vi "Connect.vi"(8 "error in (no error)":errorcluster, 10 "Session - Pipeline":path=path "Z:/users/Manolis/Labview/Scanner/sessions.dsn", 11 "Database in":refnum<class "Database.lvclass">) -> (0 "error out":errorcluster, 3 "Database out":refnum<class "Database.lvclass">)   [LabVIEW 2014, in "Database.lvclass"]
uses:
  Database.lvclass
  Database.lvclass/Database.ctl
  <vilib>/addons/database/Connection.llb/DB Tools Open Connec (Path).vi
  <vilib>/addons/database/NI_Database_API.lvlib
panel:
  in  "Session - Commons":path=path "Z:/users/Manolis/Labview/Scanner/sessions.dsn"
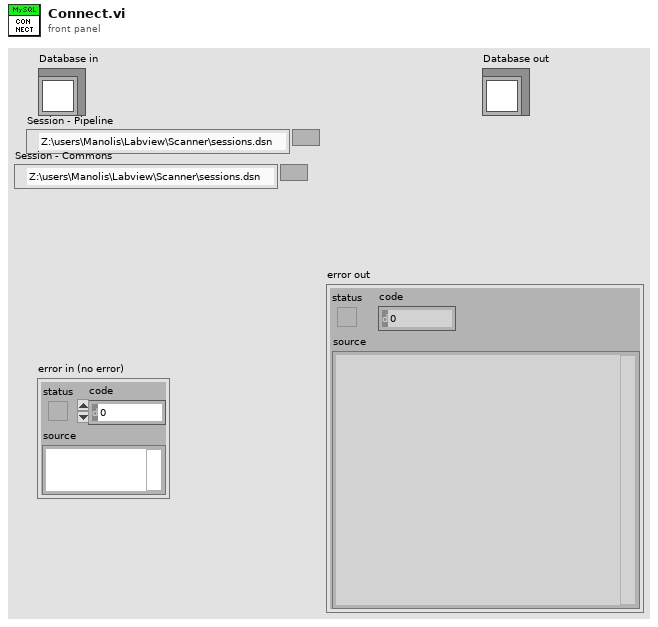
[diagram p1: front panel]
types:
  T1 = typedef "NI_Database_API.lvlib/Conn ObjectReference.ctl" = refnum<k1>
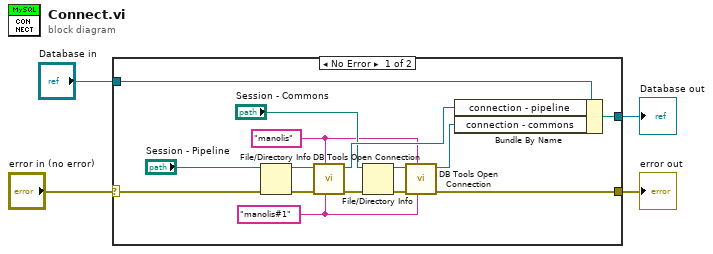
[diagram p0: block diagram]
diagram:
  n1 = case shown="No Error" "error in (no error)" {
    selector: "error in (no error)" -> [w14 w21]
    tunnel: [w7 w21] -> w3
    tunnel: [w18 w20] -> w1
    tunnel: "Database in" -> [w19 w20]
    frame No Error {
      w5 = "manolis#1" ("password")
      w6 = "manolis" ("userID")
      n2 = File/Directory Info(path="Session - Pipeline", error in=w14) -> (path out=w16:path, error out=w13:errorcluster)  [unwired: 5 out]
      n3 = call-poly <vilib>:"DB Tools Open Connection.vi"("password"=w5, "userID"=w6, "error in (no error)"=w13, "connection information"=w16) -> ("error out"=w9:errorcluster, "connection reference"=w15:T1)  [unwired: 4 in]
      n4 = File/Directory Info(path="Session - Commons", error in=w9) -> (path out=w11:path, error out=w8:errorcluster)  [unwired: 5 out]
      n5 = call-poly <vilib>:"DB Tools Open Connection.vi"("password"=w5, "userID"=w6, "error in (no error)"=w8, "connection information"=w11) -> ("error out"=w7:errorcluster, "connection reference"=w12:T1)  [unwired: 4 in]
      n6 = Bundle By Name(cluster=w19, "connection - pipeline"=w15, "connection - commons"=w12) -> (w18:refnum<class "Database.lvclass">)
    }
    frame Error {
    }
  }
  "error out" <- w3
  "Database out" <- w1
